vi "Sperical to cartesian (SubVI).vi"(6 "SinFI":dbl[](array[numeric]), 7 "Cos FI":dbl[](array[numeric]), 9 "Cos Tetta":dbl[](array[numeric]), 10 "SinTetta":dbl[](array[numeric]), 11 "Data":dbl[][](array[numeric])) -> (1 "XZ":cluster{dbl[], dbl[]}, 2 "plots out":refnum<class "Base Datatype.lvclass">[](array[class]), 3 "XY3":cluster{dbl[], dbl[]}, 4 "YZ":cluster{dbl[], dbl[]})   [LabVIEW 2015]
uses:
  <vilib>/Native 3D Graph/classes/Base Datatype.lvclass
  <vilib>/Native 3D Graph/xcontrol/3DPC_SurfacePlot.xctl
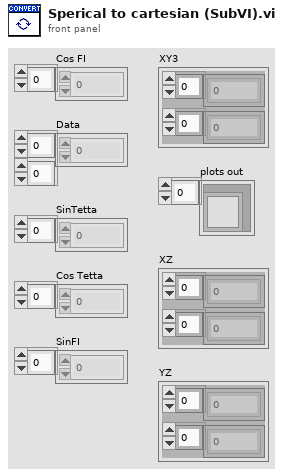
[diagram p1: front panel]
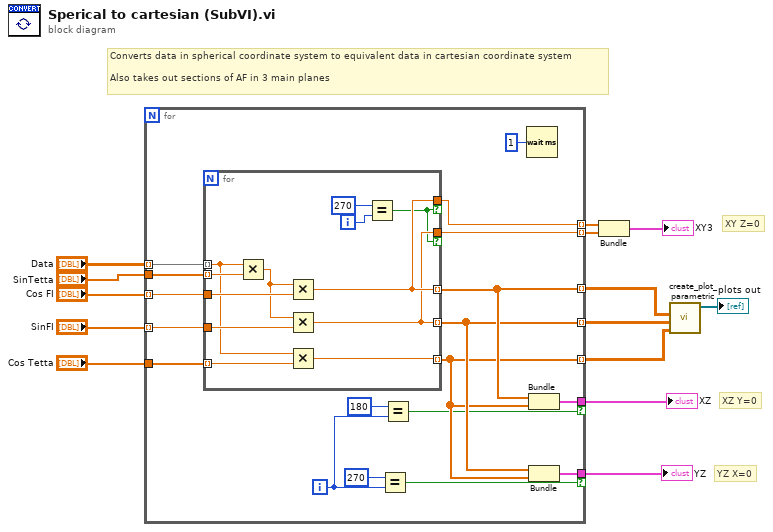
[diagram p0: block diagram]
diagram:
  # "Converts data in spherical coordinate system to equivalent data in cartesian coordinate system\n\nAlso takes out sections of AF in 3 main planes"
  # "YZ X=0"
  # "XZ Y=0"
  # "XY Z=0"
  n1 = for {
    tunnel: "Data" -> [w32] mode=indexing
    tunnel: "SinFI" -> [w31] mode=indexing
    tunnel: "Cos FI" -> [w30] mode=indexing
    tunnel: "SinTetta" -> [w29]
    tunnel: [w27] -> w5 mode=indexing
    tunnel: [w26] -> w6 mode=indexing
    tunnel: "Cos Tetta" -> [w28]
    tunnel: [w25] -> w7 mode=indexing
    tunnel: [w23] -> w12 if=w21
    tunnel: [w24] -> w13 if=w18
    tunnel: [w17] -> w9 mode=indexing
    tunnel: [w16] -> w10 mode=indexing
    i -> [w19]
    n2 = for {
      tunnel: w32 -> [w40] mode=indexing
      tunnel: w31 -> [w41]
      tunnel: w30 -> [w43]
      tunnel: w29 -> [w44] mode=indexing
      tunnel: [w35] -> w27 mode=indexing
      tunnel: [w34] -> w26 mode=indexing
      tunnel: w28 -> [w39] mode=indexing
      tunnel: [w38] -> w25 mode=indexing
      tunnel: [w35] -> w17 if=w33
      tunnel: [w34] -> w16 if=w33
      i -> [w36]
      n3 = Multiply(x=w40, y=w44) -> (x*y=w42:dbl)
      n4 = Multiply(x=w42, y=w43) -> (x*y=w35:dbl)
      n5 = Multiply(x=w42, y=w41) -> (x*y=w34:dbl)
      n6 = Multiply(x=w40, y=w39) -> (x*y=w38:dbl)
      n7 = Equal?(x=270, y=w36) -> (x = y?=w33:bool)
    }
    n8 = Equal?(x=270, y=w19) -> (x = y?=w18:bool)
    n9 = Equal?(x=180, y=w19) -> (x = y?=w21:bool)
    n10 = Wait (ms)(milliseconds to wait=u32 1) -> ()  [unwired: 1 out]
    n11 = Bundle(w27, w25) -> (w23:cluster{dbl[], dbl[]})  [unwired: 1 in]
    n12 = Bundle(w26, w25) -> (w24:cluster{dbl[], dbl[]})  [unwired: 1 in]
  }
  "YZ" <- w13
  "XZ" <- w12
  n13 = Bundle(w9, w10) -> (→"XY3":cluster{dbl[], dbl[]})  [unwired: 1 in]
  n14 = call <vilib>:"create_plot_parametric.vi"("z matrix"=w7, "y matrix"=w6, "x matrix"=w5) -> ("plots out"=→"plots out":refnum<class "Base Datatype.lvclass">[])  [unwired: 2 in, 6 out]
